vi "Init.vi"(8 "error in (no error)":errorcluster, 11 "Mock Report In":refnum<class "Mock Report.lvclass">) -> (0 "error out":errorcluster, 3 "Mock Report Out":refnum<class "Mock Report.lvclass">)   [LabVIEW 2020, in "Mock Report.lvclass"]
uses:
  Mock Report.lvclass
  C:/git/astemes-lunit/source/Framework/Report Interface/Report Interface.lvclass
  C:/git/astemes-lunit/source/Plugins/Report/Report.lvclass
  source/Plugins/Report/Report.lvclass/Report.ctl
  source/Plugins/Report Generator/Report Generator.lvclass
  source/Plugins/Report/Report.lvclass
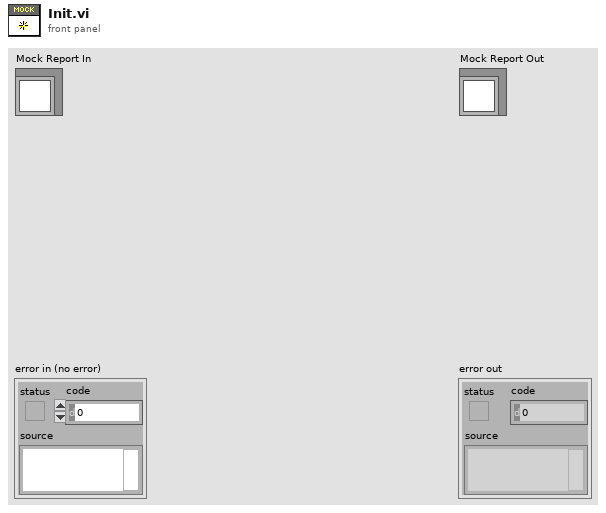
[diagram p1: front panel]
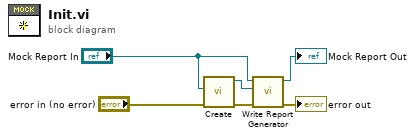
[diagram p0: block diagram]
diagram:
  n1 = call "Create.vi"("error in (no error)"="error in (no error)", "Report Interface"="Mock Report In") -> ("error out"=w6:errorcluster, "Report Generator Out"=w3:refnum<class "Report Generator.lvclass">)  [unwired: 8 in]
  n2 = call "Write Report Generator.vi"("error in (no error)"=w6, "Report Generator"=w3, "Report In"="Mock Report In") -> ("error out"=→"error out":errorcluster, "Report Out"=→"Mock Report Out":refnum<class "Mock Report.lvclass">)  [unwired: 7 in]
